vi "Query Pulse Width.vi"(4 "pulse number":i32=1 min=1 max=4, 6 "channel":i32=1 min=1 max=4, 8 "error in (no error)":errorcluster, 11 "VISA resource name":refnum<visa-resource-name>) -> (0 "error Out (no error)":errorcluster, 2 "pulse width (s)":dbl format="%^#_6g", 3 "VISA resource name out":refnum<visa-resource-name>)   [LabVIEW 2019, in "Pulse Rider PG-1000.lvlib"]
doc: "Query the pulse width for the specified pulse relative to the selected output channel.\n\nPulse Width = Period × Duty Cycle / 100. The pulse width must be less than the period. Pulse Width <= Pulse Period\n\nw: the pulse width in second\nchannel: the output channel int from 1 to 4\npulse_nb: the pulse number int from 1 to 4"
uses:
  <instrlib>/Pulse Rider PG-1000/Pulse Rider PG-1000.lvlib
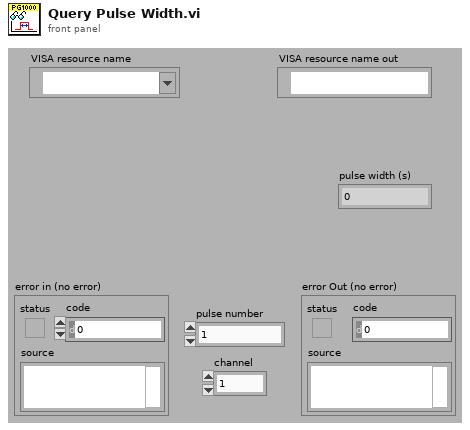
[diagram p1: front panel]
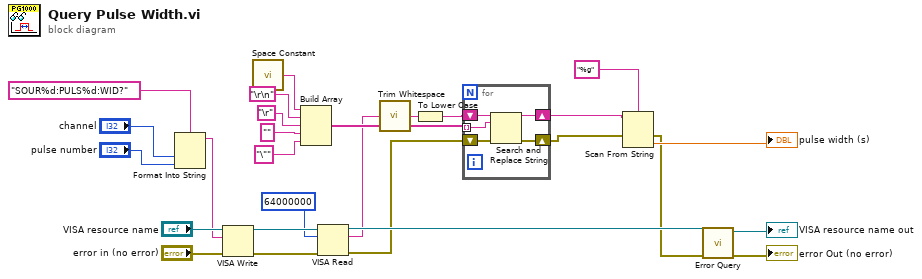
[diagram p0: block diagram]
diagram:
  n1 = Format Into String(format string="SOUR%d:PULS%d:WID?", "channel", "pulse number") -> (resulting string=w8:string)  [unwired: 2 in, 1 out]
  n2 = VISA Write(VISA resource name="VISA resource name", write buffer=w8, error in (no error)="error in (no error)") -> (VISA resource name out=w23:refnum<visa-resource-name>, error out=w22:errorcluster)  [unwired: 1 out]
  n3 = call <vilib>:"Space Constant.vi"() -> ("String"=w19:string)
  n4 = Build Array(w19, "\r\n", "\r", "", "\"") -> (w14:string[])
  n5 = VISA Read(VISA resource name=w23, byte count=u32 64000000, error in (no error)=w22) -> (VISA resource name out=w20:refnum<visa-resource-name>, read buffer=w12:string, error out=w3:errorcluster)  [unwired: 1 out]
  n6 = call <vilib>:"Trim Whitespace.vi"("string"=w12) -> ("trimmed string"=w13:string)  [unwired: 1 in]
  n7 = To Lower Case(string=w13) -> (all lower case string=w11:string)
  n8 = for {
    tunnel: w14 -> [w30] mode=indexing
    shift-right: [w32] -> w7
    shift-left: w11 -> [w31]
    shift-right: [w28] -> w2
    shift-left: w3 -> [w29]
    n9 = Search and Replace String(input string=w31, search string=w30, error in=w29) -> (result string=w32:string, error out=w28:errorcluster)  [unwired: 5 in, 2 out]
  }
  n10 = Scan From String(format string="%g", input string=w7, error in=w2) -> (error out=w1:errorcluster, output 1=→"pulse width (s)":dbl)  [unwired: 2 in, 2 out]
  n11 = call <instrlib>:"Error Query.vi"("error in (no error)"=w1, "VISA resource name"=w20) -> ("error out"=→"error Out (no error)":errorcluster, "VISA resource name out"=→"VISA resource name out":refnum<visa-resource-name>)  [unwired: 6 in, 2 out]
